vi "CgHardware.vi"() -> ()   [LabVIEW 2009]
uses:
  <vilib>/Instr/_visa.llb/VISA Configure Serial Port (Instr).vi
  GlobalVariables.vi
  Cyberglove SubVIs/Hardware/HCalSet.vi
  Cyberglove SubVIs/Hardware/HCalGet.vi
panel:
  out "Min":u8[](array[numeric])
  out "Max":u8[](array[numeric])
  in  "Reset":bool
  out "Hardware Calibration":u8[][](array[numeric])
  in  "Set Current":bool
  in  "Revert":bool
  in  "Load Current":bool
  out "Raw Data":u8[](array[numeric])
  in  "stop":bool
  in  "Offset":u8=1 min=1 step=1
  in  "Gain":u8=1 min=1 step=1
  out "Sensor Value":u8
  out "Hand":string
  in  "Sensor Selection":T1(radio)
  in  "Cyberglove COM Port":refnum<visa-resource-name>="COM1"
  out "Sensor Names":string[](array[string])
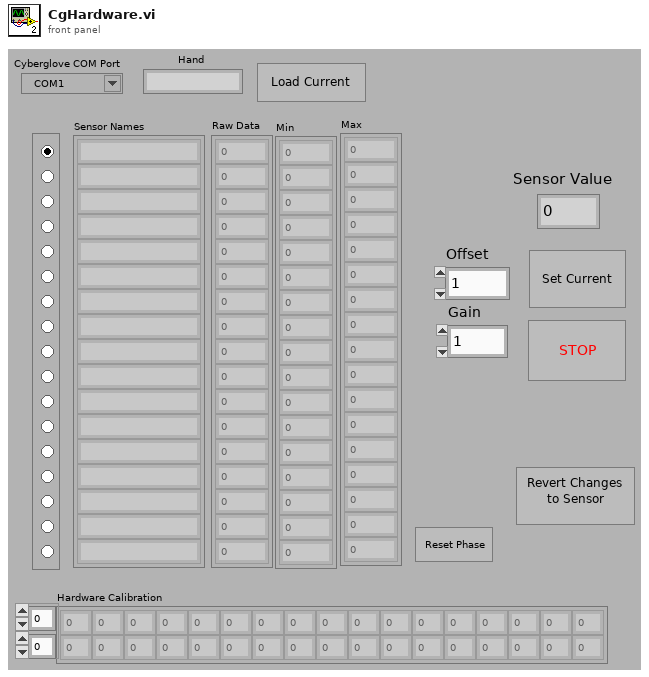
[diagram p1: front panel]
types:
  T1 = enum32{"Radio Selection 1", "Radio Selection 2", "Radio Selection 3", "Radio Selection 4", "Radio Selection 5", "Radio Selection 6", "Radio Selection 7", "Radio Selection 8", "Radio Selection 9", "Radio Selection 10", "Radio Selection 11", "Radio Selection 12", "Radio Selection 13", "Radio Selection 14", "Radio Selection 15", "Radio Selection 16", "Radio Selection 17", "Radio Selection 18", "Radio Selection 19", "Radio Selection 20"}
  T2 = typedef "Semaphore RefNum" = refnum<k1>
  T3 = typedef "eventvkey.ctl" = enum16{"ASCII", "Enter", "Return", "Shift", "Ctrl", "Alt", "Cmd", "Opt", "Caps", "NumLock", "Clear", "Break", "Up", "Down", "Left", "Right", "Insert", "Delete", "Home", "End", "PageUp", "PageDown", "Escape", "Help", "Pause", "ScrollLock", "F1", "F2", "F3", "F4", "F5", "F6", "F7", "F8", "F9", "F10", "F11", "F12", "F13", "F14", "F15", "F16", "F17", "F18", "F19", "F20", "F21", "F22", "F23", "F24", "Play", "VolumeUp", "VolumeDown", "Mute", "Two Byte Char"}
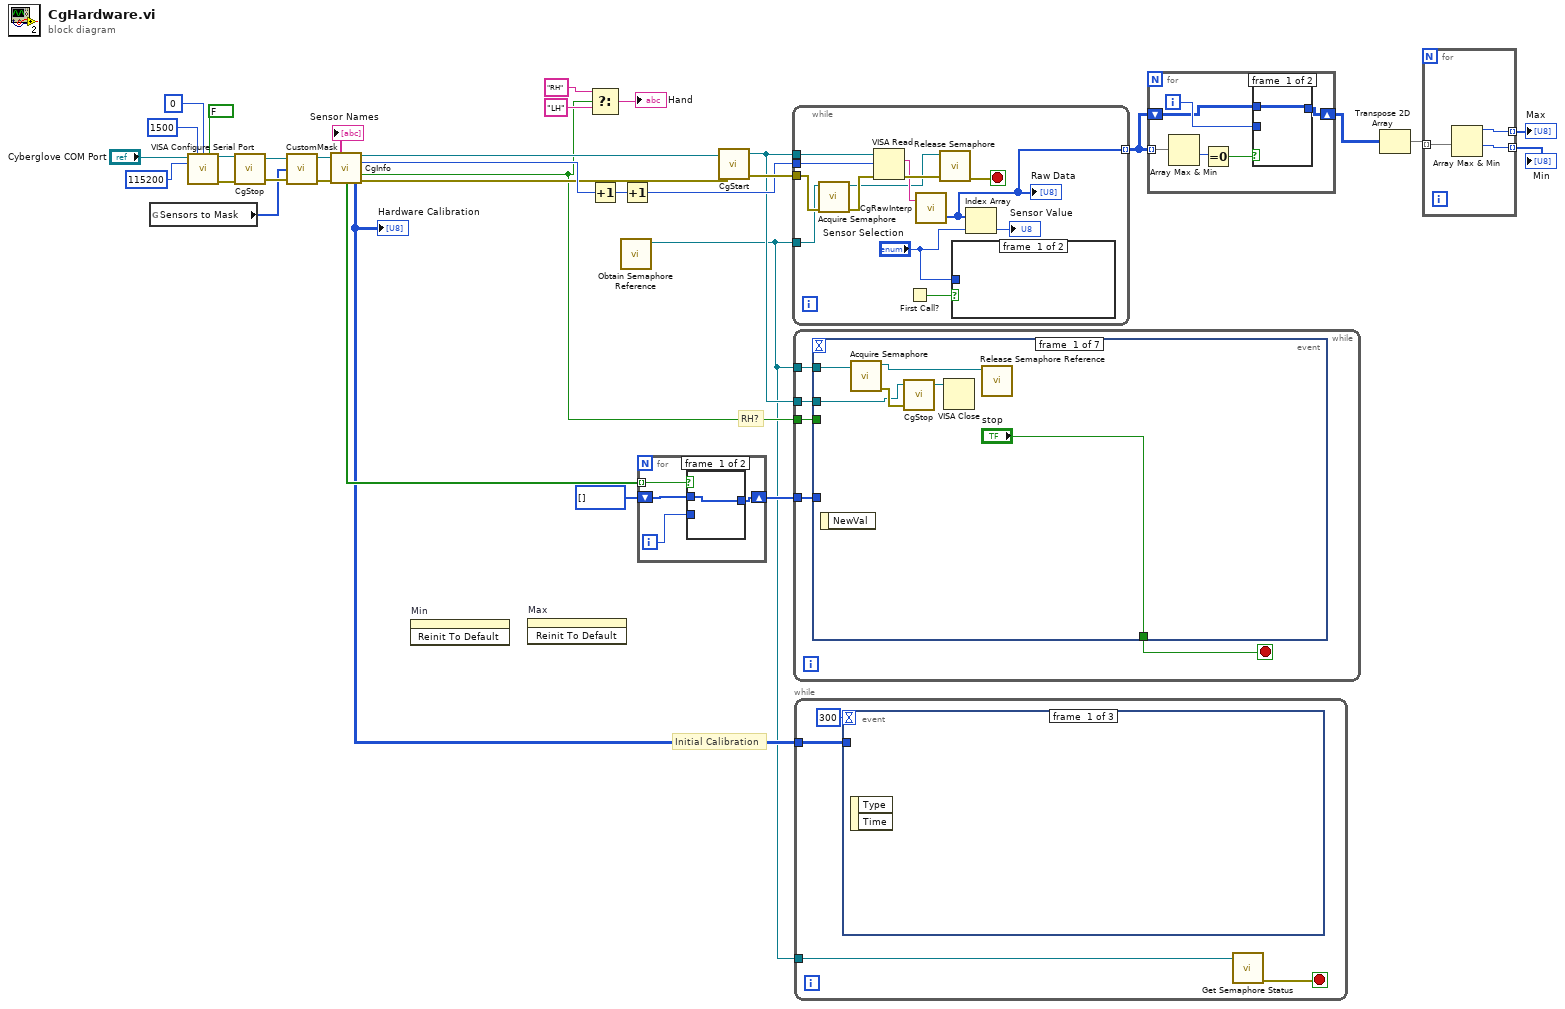
[diagram p0: block diagram]
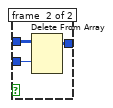
[diagram p2: hidden frame]
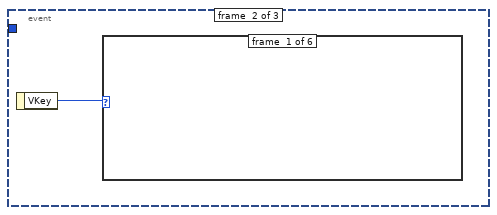
[diagram p3: hidden frame]
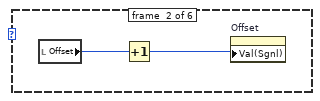
[diagram p4: hidden frame]
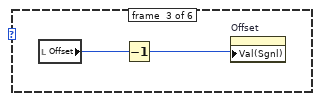
[diagram p5: hidden frame]
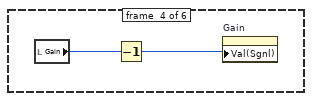
[diagram p6: hidden frame]
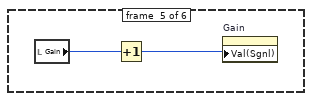
[diagram p7: hidden frame]
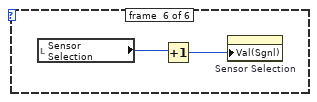
[diagram p8: hidden frame]
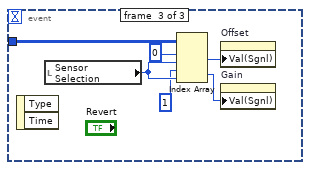
[diagram p9: hidden frame]
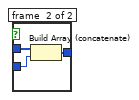
[diagram p10: hidden frame]
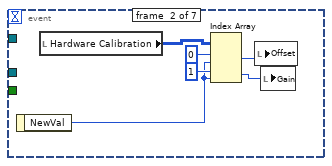
[diagram p11: hidden frame]
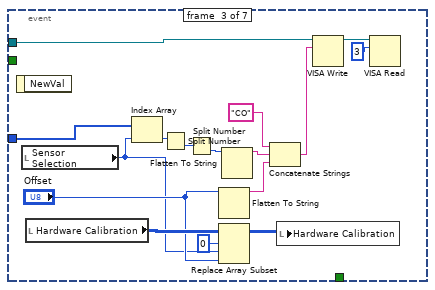
[diagram p12: hidden frame]
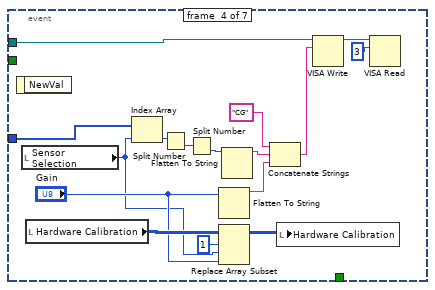
[diagram p13: hidden frame]
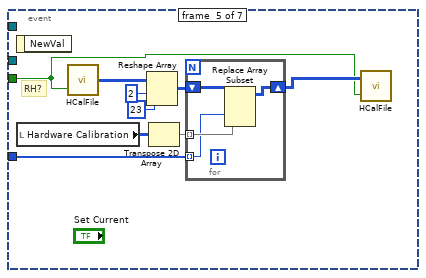
[diagram p14: hidden frame]
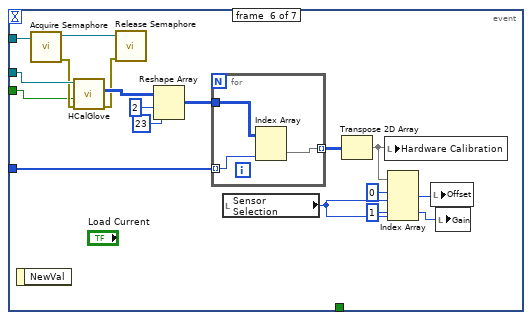
[diagram p15: hidden frame]
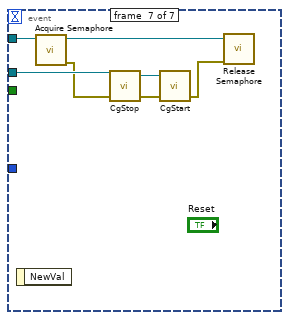
[diagram p16: hidden frame]
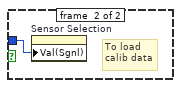
[diagram p17: hidden frame]
diagram:
  # "Initial Calibration"
  # "RH?"
  n1 = global read "GlobalVariables.vi" "Sensors to Mask"() -> (w9:u32[])
  n2 = call-poly "VISA Configure Serial Port"("VISA resource name"="Cyberglove COM Port", "timeout (10sec)"=u32 1500, "termination char\n(0xA = '\\n' = LF)"=u8 0 ("termination char\n(0xA = '\\n' = LF)"), "Enable Termination\nChar (T)"=FALSE ("Enable Termination\nChar (T)"), "baud rate (9600)"=u32 115200) -> ("VISA resource name out"=w30:refnum<visa-resource-name>, "error out"=w29:errorcluster)  [unwired: 9 in]
  n3 = call "CgStop.vi"("error in (no error)"=w29, "VISA resource name"=w30) -> ("error out"=w28:errorcluster, "VISA resource name out"=w27:refnum<visa-resource-name>)  [unwired: 2 in]
  n4 = call "CustomMask.vi"("error in (no error)"=w28, "Custom Mask"=w9, "VISA resource name"=w27) -> ("error out"=w24:errorcluster, "VISA resource name out"=w25:refnum<visa-resource-name>)
  n5 = call "CgInfo.vi"("VISA resource name"=w25, "error in (no error)"=w24) -> ("VISA resource name out"=w13:refnum<visa-resource-name>, "#Sensors"=w20:i32, "RH?"=w8:bool, "Sensor Names"=→"Sensor Names":string[], "Sensors Active"=w16:bool[], "Hardware Calibration"=w7:u8[][], "error out"=w12:errorcluster)  [unwired: 7 in]
  "Hardware Calibration" <- w7
  n6 = invoke on="Min" class="Arr (strict)" method="Reinit To Default"() -> ()  [unwired: 3 in, 3 out]
  n7 = invoke on="Max" class="Arr (strict)" method="Reinit To Default"() -> ()  [unwired: 3 in, 3 out]
  n8 = Select(t="RH" ("Window Title (\"\")"), s=w8, f="LH" ("Window Title (\"\")")) -> (s? t:f=→"Hand":string)
  n9 = Increment(x=w20) -> (x+1=w19:i32)
  n10 = call <vilib>:"Obtain Semaphore Reference.vi"() -> ("semaphore"=w6:T2)  [unwired: 5 in, 2 out]
  n11 = Increment(x=w19) -> (x+1=w17:i32)
  n12 = for {
    tunnel: w16 -> [w38] mode=indexing
    shift-right: [w35] -> w10
    shift-left: u8[] [] -> [w36]
    i -> [w37]
    n13 = case shown="True" w38 {
      tunnel: w37 -> [_ w40]
      tunnel: [w39 w42] -> w35
      tunnel: w36 -> [w39 w41]
      frame #0 {
      }
      frame #1 {
        n14 = Build Array (concatenate)(w41, w40) -> (w42:i32[])
      }
    }
  }
  n15 = call "CgStart.vi"("error in (no error)"=w12, "VISA resource name"=w13) -> ("error out"=w18:errorcluster, "VISA resource name out"=w14:refnum<visa-resource-name>)  [unwired: 2 in]
  n16 = while {
    tunnel: w14 -> [w52]
    tunnel: w18 -> [w55]
    tunnel: w6 -> [w54]
    tunnel: w17 -> [w50]
    tunnel: [w43] -> w3 mode=indexing
    stop <- w46 stop-if-true
    n17 = call <vilib>:"Acquire Semaphore.vi"("error in (no error)"=w55, "semaphore"=w54) -> ("error out"=w53:errorcluster, "semaphore out"=w47:T2)  [unwired: 3 in, 1 out]
    n18 = VISA Read(VISA resource name=w52, byte count=w50, error in (no error)=w53) -> (read buffer=w49:string, error out=w51:errorcluster)  [unwired: 2 out]
    n19 = First Call?() -> (First Call?: T/F=w45:bool)
    n20 = call "CgRawInterp.vi"("Cyberglove Out"=w49) -> ("Raw Data"=w43:u8[])  [unwired: 1 in, 1 out]
    "Raw Data" <- w43
    n21 = call <vilib>:"Release Semaphore.vi"("error in (no error)"=w51, "semaphore"=w47) -> ("error out"=w46:errorcluster)  [unwired: 4 in, 1 out]
    n22 = case shown="True" w45 {
      tunnel: "Sensor Selection" -> [_ w56]
      frame #0 {
      }
      frame #1 {
        # "To load\ncalib data"
        n23 = property on="Sensor Selection" class="RadioBtnsControl (strict)"("Val(Sgnl)"=w56) -> ()  [unwired: 2 in, 2 out]
      }
    }
    n24 = Index Array(array=w43, index="Sensor Selection") -> (element=→"Sensor Value":u8)
  }
  n25 = while {
    tunnel: w6 -> [w61]
    tunnel: w14 -> [w60]
    tunnel: w10 -> [w58]
    tunnel: w8 -> [w57]
    stop <- w59 stop-if-true
    n26 = event shown="[5] \"Load Current\": Value Change" {
      selector: _ -> [_ _ _ _ _ _ _]
      dyn-events: _ -> [_ _ _ _ _ _ _]
      timeout: _ -> [_ _ _ _ _ _ _]
      tunnel: w61 -> [w67 _ _ _ _ w123 w146]
      tunnel: w60 -> [w65 _ w89 w105 _ w131 w145]
      tunnel: ["stop" _ _ _ _ _ _] -> w59
      tunnel: w58 -> [_ _ w88 w104 w114 w133 _]
      tunnel: w57 -> [_ _ _ _ w110 w119 _]
      event #0 {
        n27 = event-data() -> ()  [unwired: 1 in, 1 out]
        n28 = call <vilib>:"Acquire Semaphore.vi"("semaphore"=w67) -> ("error out"=w66:errorcluster, "semaphore out"=w63:T2)  [unwired: 4 in, 1 out]
        n29 = call "CgStop.vi"("error in (no error)"=w66, "VISA resource name"=w65) -> ("VISA resource name out"=w62:refnum<visa-resource-name>)  [unwired: 2 in, 1 out]
        n30 = VISA Close(VISA resource name=w62) -> ()  [unwired: 1 in, 1 out]
        n31 = call <vilib>:"Release Semaphore Reference.vi"("semaphore"=w63) -> ()  [unwired: 9 in, 2 out]
      }
      event #1 {
        n32 = event-data() -> ("NewVal"=w69:T1)  [unwired: 1 in]
        n33 = local read "Hardware Calibration"() -> (w68:u8[][])
        n34 = Index Array(array=w68, index (row) #1=0 ("disabled index (row)"), index (col) #1=w69, index (row) #2=1 ("disabled index (row)"), index (col) #2=w69) -> (element #1=w71:u8, element #2=w70:u8)
        n35 = local write "Offset"(w71) -> ()
        n36 = local write "Gain"(w70) -> ()
      }
      event #2 {
        n37 = event-data() -> ()  [unwired: 1 in, 1 out]
        n38 = local read "Sensor Selection"() -> (w77:T1)
        n39 = local read "Hardware Calibration"() -> (w79:u8[][])
        n40 = Index Array(array=w88, index=w77) -> (element=w81:i32)
        n41 = Split Number(x=w81) -> (lo(x)=w82:u16)  [unwired: 1 out]
        n42 = Split Number(x=w82) -> (lo(x)=w80:u8)  [unwired: 1 out]
        n43 = Flatten To String(anything="Offset") -> (data string=w86:string)  [unwired: 3 in, 2 out]
        n44 = Replace Array Subset(array=w79, new element="Offset", index (row)=0 ("disabled index (row)"), index (col)=w77) -> (w75:u8[][])
        n45 = Flatten To String(anything=w80) -> (data string=w87:string)  [unwired: 3 in, 2 out]
        n46 = Concatenate Strings("CO" ("string"), w87, w86) -> (w74:string)
        n47 = local write "Hardware Calibration"(w75) -> ()
        n48 = VISA Write(VISA resource name=w89, write buffer=w74) -> (VISA resource name out=w84:refnum<visa-resource-name>)  [unwired: 1 in, 2 out]
        n49 = VISA Read(VISA resource name=w84, byte count=u32 3) -> ()  [unwired: 1 in, 4 out]
      }
      event #3 {
        n50 = event-data() -> ()  [unwired: 1 in, 1 out]
        n51 = local read "Sensor Selection"() -> (w91:T1)
        n52 = local read "Hardware Calibration"() -> (w94:u8[][])
        n53 = Index Array(array=w104, index=w91) -> (element=w96:i32)
        n54 = Split Number(x=w96) -> (lo(x)=w97:u16)  [unwired: 1 out]
        n55 = Split Number(x=w97) -> (lo(x)=w95:u8)  [unwired: 1 out]
        n56 = Flatten To String(anything="Gain") -> (data string=w102:string)  [unwired: 3 in, 2 out]
        n57 = Replace Array Subset(array=w94, new element="Gain", index (row)=1 ("disabled index (row)"), index (col)=w91) -> (w90:u8[][])
        n58 = Flatten To String(anything=w95) -> (data string=w103:string)  [unwired: 3 in, 2 out]
        n59 = Concatenate Strings("CG" ("string"), w103, w102) -> (w100:string)
        n60 = local write "Hardware Calibration"(w90) -> ()
        n61 = VISA Write(VISA resource name=w105, write buffer=w100) -> (VISA resource name out=w99:refnum<visa-resource-name>)  [unwired: 1 in, 2 out]
        n62 = VISA Read(VISA resource name=w99, byte count=u32 3) -> ()  [unwired: 1 in, 4 out]
      }
      event #4 {
        # "RH?"
        n63 = event-data() -> ()  [unwired: 1 in, 1 out]
        n64 = local read "Hardware Calibration"() -> (w113:u8[][])
        n65 = call-poly "HCalFile.vi"("RH?"=w110) -> ("Calibration Array"=w109:u8[][])  [unwired: 1 in]
        n66 = Reshape Array(w109, 2 ("dimension size"), 23 ("dimension size")) -> (w108:u8[][])
        n67 = Transpose 2D Array(2D array=w113) -> (transposed array=w112:u8[][])
        n68 = for {
          tunnel: w114 -> [w115] mode=indexing
          shift-right: [w116] -> w111
          shift-left: w108 -> [w118]
          tunnel: w112 -> [w117] mode=indexing
          n69 = Replace Array Subset(array=w118, new element=w117, index (col)=w115) -> (w116:u8[][])  [unwired: 1 in]
        }
        n70 = call-poly "HCalFile.vi"("RH?"=w110, "Calibration In"=w111) -> ()  [unwired: 1 out]
      }
      event #5 {
        n71 = event-data() -> ()  [unwired: 1 in, 1 out]
        n72 = call <vilib>:"Acquire Semaphore.vi"("semaphore"=w123) -> ("error out"=w122:errorcluster, "semaphore out"=w120:T2)  [unwired: 4 in, 1 out]
        n73 = call "HCalGlove.vi"("error in (no error)"=w122, "RH?"=w119, "VISA Resource In"=w131) -> ("error out"=w121:errorcluster, "Calibration Array"=w136:u8[][])  [unwired: 2 in, 1 out]
        n74 = call <vilib>:"Release Semaphore.vi"("error in (no error)"=w121, "semaphore"=w120) -> ()  [unwired: 4 in, 2 out]
        n75 = Reshape Array(w136, 2 ("dimension size"), 23 ("dimension size")) -> (w132:u8[][])
        n76 = for {
          tunnel: w133 -> [w137] mode=indexing
          tunnel: w132 -> [w139]
          tunnel: [w138] -> w130 mode=indexing
          n77 = Index Array(array=w139, index (col)=w137) -> (element=w138:u8[])  [unwired: 1 in]
        }
        n78 = local read "Sensor Selection"() -> (w128:T1)
        n79 = Transpose 2D Array(2D array=w130) -> (transposed array=w129:u8[][])
        n80 = local write "Hardware Calibration"(w129) -> ()
        n81 = Index Array(array=w129, index (row) #1=0 ("disabled index (row)"), index (col) #1=w128, index (row) #2=1 ("disabled index (row)"), index (col) #2=w128) -> (element #1=w125:u8, element #2=w124:u8)
        n82 = local write "Offset"(w125) -> ()
        n83 = local write "Gain"(w124) -> ()
      }
      event #6 {
        n84 = event-data() -> ()  [unwired: 1 in, 1 out]
        n85 = call <vilib>:"Acquire Semaphore.vi"("semaphore"=w146) -> ("error out"=w144:errorcluster, "semaphore out"=w141:T2)  [unwired: 4 in, 1 out]
        n86 = call "CgStop.vi"("error in (no error)"=w144, "VISA resource name"=w145) -> ("error out"=w142:errorcluster, "VISA resource name out"=w143:refnum<visa-resource-name>)  [unwired: 2 in]
        n87 = call "CgStart.vi"("error in (no error)"=w142, "VISA resource name"=w143) -> ("error out"=w140:errorcluster)  [unwired: 2 in, 1 out]
        n88 = call <vilib>:"Release Semaphore.vi"("error in (no error)"=w140, "semaphore"=w141) -> ()  [unwired: 4 in, 2 out]
      }
    }
  }
  n89 = while {
    tunnel: w7 -> [w150]
    tunnel: w6 -> [w147]
    stop <- w148 stop-if-true
    n90 = event shown="[1] Key Down" {
      selector: _ -> [_ _ _]
      dyn-events: _ -> [_ _ _]
      timeout: 300 -> [_ _ _]
      tunnel: w150 -> [_ _ w167]
      event #0 {
        n91 = event-data() -> ()  [unwired: 1 in, 2 out]
      }
      event #1 {
        n92 = event-data() -> ("VKey"=w151:T3)  [unwired: 1 in]
        n93 = case shown="\"Return\"" w151 {
          frame #0 {
          }
          frame #1 {
            n94 = local read "Offset"() -> (w153:u8)
            n95 = Increment(x=w153) -> (x+1=w152:u8)
            n96 = property on="Offset" class="DigNum (strict)"("Val(Sgnl)"=w152) -> ()  [unwired: 2 in, 2 out]
          }
          frame #2 {
            n97 = local read "Offset"() -> (w155:u8)
            n98 = Decrement(x=w155) -> (x-1=w154:u8)
            n99 = property on="Offset" class="DigNum (strict)"("Val(Sgnl)"=w154) -> ()  [unwired: 2 in, 2 out]
          }
          frame #3 {
            n100 = local read "Gain"() -> (w157:u8)
            n101 = Decrement(x=w157) -> (x-1=w156:u8)
            n102 = property on="Gain" class="DigNum (strict)"("Val(Sgnl)"=w156) -> ()  [unwired: 2 in, 2 out]
          }
          frame #4 {
            n103 = local read "Gain"() -> (w159:u8)
            n104 = Increment(x=w159) -> (x+1=w158:u8)
            n105 = property on="Gain" class="DigNum (strict)"("Val(Sgnl)"=w158) -> ()  [unwired: 2 in, 2 out]
          }
          frame #5 {
            n106 = local read "Sensor Selection"() -> (w161:T1)
            n107 = Increment(x=w161) -> (x+1=w160:T1)
            n108 = property on="Sensor Selection" class="RadioBtnsControl (strict)"("Val(Sgnl)"=w160) -> ()  [unwired: 2 in, 2 out]
          }
        }
      }
      event #2 {
        n109 = event-data() -> ()  [unwired: 1 in, 2 out]
        n110 = local read "Sensor Selection"() -> (w166:T1)
        n111 = Index Array(array=w167, index (row) #1=0 ("disabled index (row)"), index (col) #1=w166, index (row) #2=1 ("disabled index (row)"), index (col) #2=w166) -> (element #1=w163:u8, element #2=w162:u8)
        n112 = property on="Offset" class="DigNum (strict)"("Val(Sgnl)"=w163) -> ()  [unwired: 2 in, 2 out]
        n113 = property on="Gain" class="DigNum (strict)"("Val(Sgnl)"=w162) -> ()  [unwired: 2 in, 2 out]
      }
    }
    n114 = call <vilib>:"Get Semaphore Status.vi"("semaphore"=w147) -> ("error out"=w148:errorcluster)  [unwired: 5 in, 5 out]
  }
  n115 = for {
    tunnel: w3 -> [w173] mode=indexing
    shift-right: [w169] -> w1
    shift-left: w3 -> [w170]
    i -> [w171]
    n116 = Array Max & Min(array=w173) -> (min value=w172:u8)  [unwired: 3 out]
    n117 = Equal To 0?(x=w172) -> (x = 0?=w168:bool)
    n118 = case shown="False" w168 {
      tunnel: w171 -> [_ w177]
      tunnel: w170 -> [w174 w176]
      tunnel: [w174 w175] -> w169
      frame #0 {
      }
      frame #1 {
        n119 = Delete From Array(array=w176, index (row)=w177) -> (array with subset deleted=w175:u8[][])  [unwired: 2 in, 1 out]
      }
    }
  }
  n120 = Transpose 2D Array(2D array=w1) -> (transposed array=w2:u8[][])
  n121 = for {
    tunnel: w2 -> [w180] mode=indexing
    tunnel: [w179] -> w5 mode=indexing
    tunnel: [w178] -> w4 mode=indexing
    n122 = Array Max & Min(array=w180) -> (max value=w179:u8, min value=w178:u8)  [unwired: 2 out]
  }
  "Max" <- w5
  "Min" <- w4
